vi "esdaq_demo.vi"() -> ()   [LabVIEW 2019]
panel:
  out "esdaqErrorOut":errorcluster
  out "DO_Array":bool[](array[boolean])
  in  "COM Status":bool
  in  "COM Port":refnum<visa-resource-name>
  in  "DIO_Array":T1(array[cluster])
  in  "AO_Array":T2(array[cluster])
  out "AI_Array":T3(array[cluster])
  # "ESDAQ-Data Acquisition System-13 DIO, 8 AI, 2 AO"
  # "Interactive Control Panel"
  # "https://github.com/enginsubasi/esdaqsys"
  # "https://github.com/enginsubasi/esdaqsys/wiki"
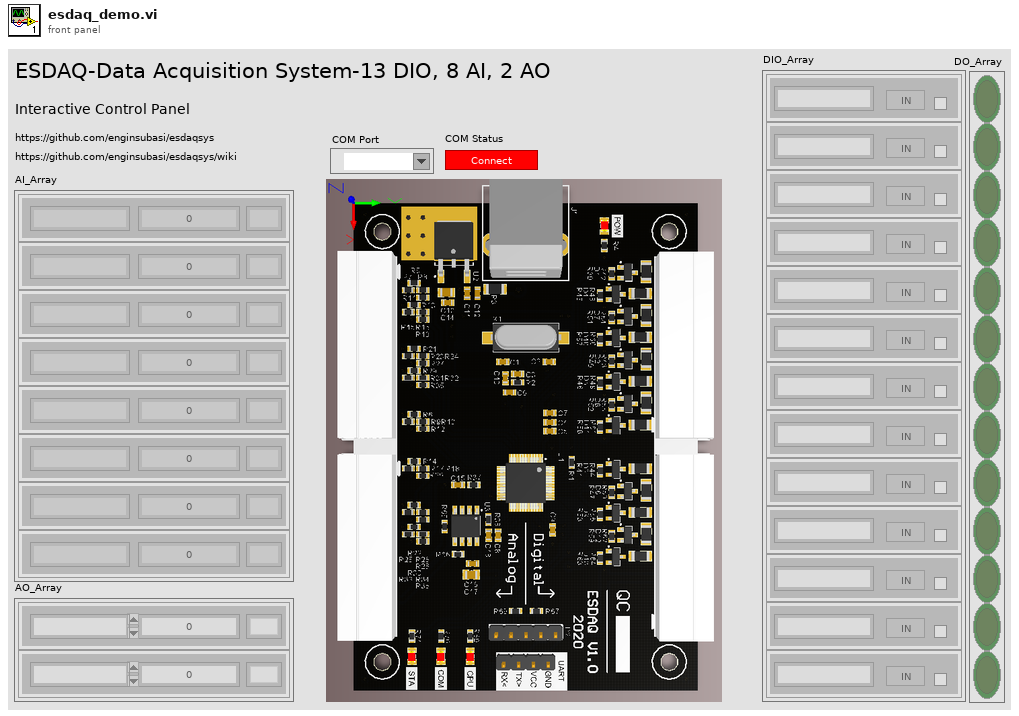
[diagram p1: front panel]
types:
  T1 = cluster{"Channel":string, "Direction":bool, "Drive":bool}[]
  T2 = cluster{"Value":u32, "Channel":string, "Unit":string}[]
  T3 = cluster{"Value":i32, "Channel":string, "Unit":string}[]
  T4 = cluster{"Value":i32, "Channel":string, "Unit":string}
  T5 = cluster{"Channel":bool, "Direction":bool, "Drive":bool}[]
  T6 = cluster{"Channel":string, "Direction":bool, "Drive":bool}
  T7 = cluster{"Value":bool, "Channel":bool, "Unit":bool}[]
  T8 = cluster{"Value":u32, "Channel":string, "Unit":string}
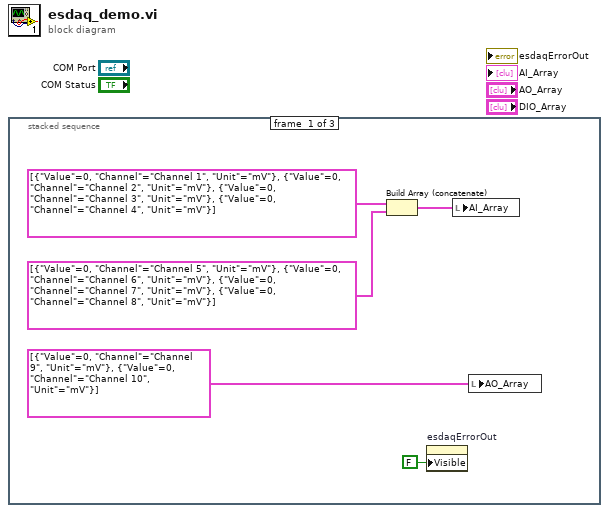
[diagram p0: block diagram]
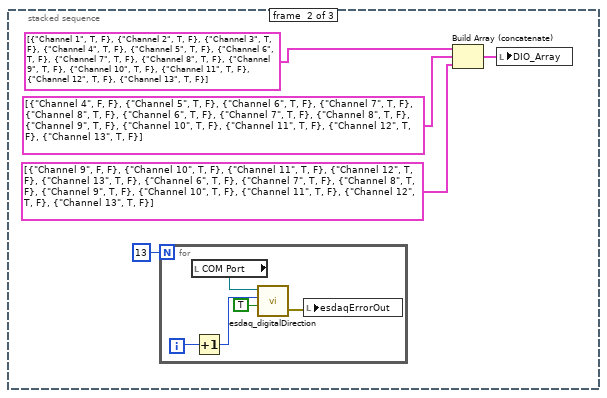
[diagram p2: hidden frame]
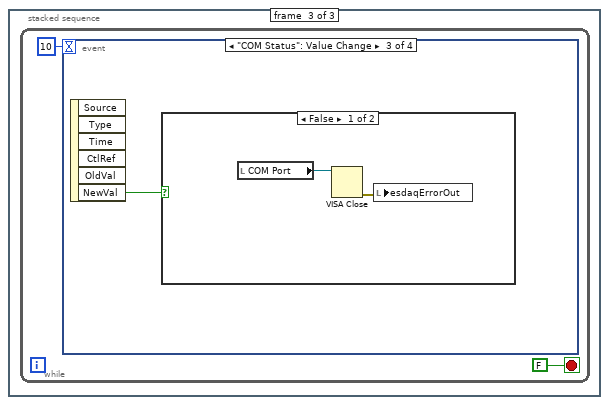
[diagram p3: hidden frame]
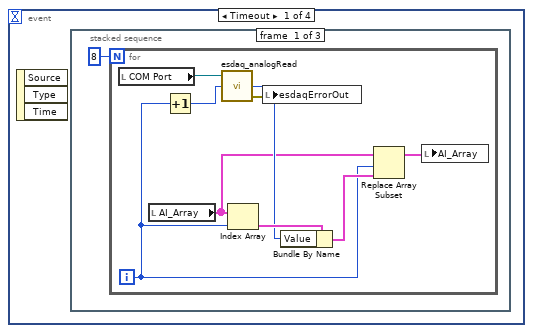
[diagram p4: hidden frame]
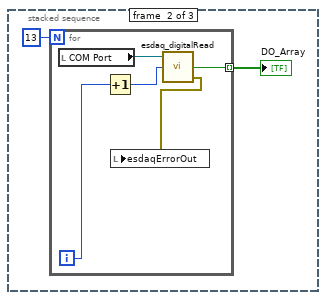
[diagram p5: hidden frame]
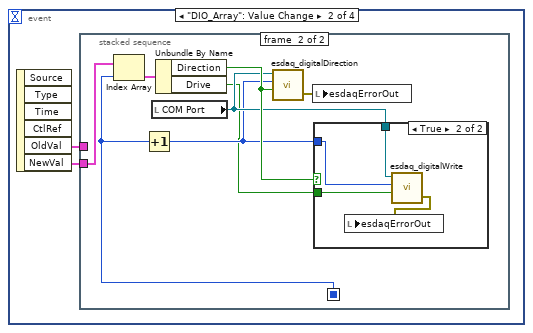
[diagram p7: hidden frame]
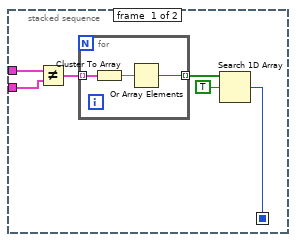
[diagram p8: hidden frame]
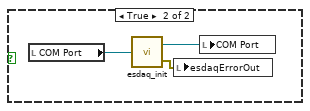
[diagram p10: hidden frame]
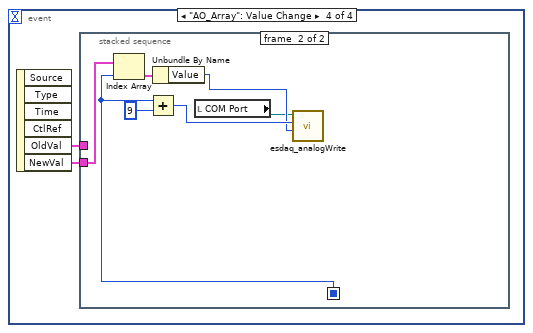
[diagram p11: hidden frame]
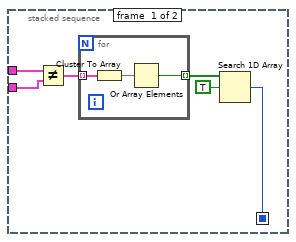
[diagram p12: hidden frame]
diagram:
  n1 = stacked-sequence {
    frame #0 {
      n2 = Build Array (concatenate)(T3 [{"Value"=0, "Channel"="Channel 1", "Unit"="mV"}, {"Value"=0, "Channel"="Channel 2", "Unit"="mV"}, {"Value"=0, "Channel"="Channel 3", "Unit"="mV"}, {"Value"=0, "Channel"="Channel 4", "Unit"="mV"}] ("AI_Array"), T3 [{"Value"=0, "Channel"="Channel 5", "Unit"="mV"}, {"Value"=0, "Channel"="Channel 6", "Unit"="mV"}, {"Value"=0, "Channel"="Channel 7", "Unit"="mV"}, {"Value"=0, "Channel"="Channel 8", "Unit"="mV"}] ("AI_Array")) -> (w3:T3)
      n3 = property on="esdaqErrorOut" class="Clust (strict)"("Visible"=FALSE) -> ()  [unwired: 2 in, 2 out]
      n4 = local write "AI_Array"(w3) -> ()
      n5 = local write "AO_Array"(T2 [{"Value"=0, "Channel"="Channel 9", "Unit"="mV"}, {"Value"=0, "Channel"="Channel 10", "Unit"="mV"}] ("AO_Array")) -> ()
    }
    frame #1 {
      n6 = for {
        N: 13 -> [_]
        i -> [w15]
        n7 = local read "COM Port"() -> (w12:refnum<visa-resource-name>)
        n8 = Increment(x=w15) -> (x+1=w14:i32)
        n9 = call "esdaq_digitalDirection.vi"("Value"=TRUE, "Channel"=w14, "esdaqPortInp"=w12) -> ("esdaqErrorOut"=w11:errorcluster)  [unwired: 1 in, 1 out]
        n10 = local write "esdaqErrorOut"(w11) -> ()
      }
      n11 = Build Array (concatenate)(T1 [{"Channel"="Channel 1", "Direction"=TRUE, "Drive"=FALSE}, {"Channel"="Channel 2", "Direction"=TRUE, "Drive"=FALSE}, {"Channel"="Channel 3", "Direction"=TRUE, "Drive"=FALSE}, {"Channel"="Channel 4", "Direction"=TRUE, "Drive"=FALSE}, {"Channel"="Channel 5", "Direction"=TRUE, "Drive"=FALSE}, {"Channel"="Channel 6", "Direction"=TRUE, "Drive"=FALSE}, {"Channel"="Channel 7", "Direction"=TRUE, "Drive"=FALSE}, {"Channel"="Channel 8", "Direction"=TRUE, "Drive"=FALSE}, {"Channel"="Channel 9", "Direction"=TRUE, "Drive"=FALSE}, {"Channel"="Channel 10", "Direction"=TRUE, "Drive"=FALSE}, {"Channel"="Channel 11", "Direction"=TRUE, "Drive"=FALSE}, {"Channel"="Channel 12", "Direction"=TRUE, "Drive"=FALSE}, {"Channel"="Channel 13", "Direction"=TRUE, "Drive"=FALSE}] ("DIO_Array"), T1 [{"Channel"="Channel 4", "Direction"=FALSE, "Drive"=FALSE}, {"Channel"="Channel 5", "Direction"=TRUE, "Drive"=FALSE}, {"Channel"="Channel 6", "Direction"=TRUE, "Drive"=FALSE}, {"Channel"="Channel 7", "Direction"=TRUE, "Drive"=FALSE}, {"Channel"="Channel 8", "Direction"=TRUE, "Drive"=FALSE}, {"Channel"="Channel 6", "Direction"=TRUE, "Drive"=FALSE}, {"Channel"="Channel 7", "Direction"=TRUE, "Drive"=FALSE}, {"Channel"="Channel 8", "Direction"=TRUE, "Drive"=FALSE}, {"Channel"="Channel 9", "Direction"=TRUE, "Drive"=FALSE}, {"Channel"="Channel 10", "Direction"=TRUE, "Drive"=FALSE}, {"Channel"="Channel 11", "Direction"=TRUE, "Drive"=FALSE}, {"Channel"="Channel 12", "Direction"=TRUE, "Drive"=FALSE}, {"Channel"="Channel 13", "Direction"=TRUE, "Drive"=FALSE}] ("DIO_Array"), T1 [{"Channel"="Channel 9", "Direction"=FALSE, "Drive"=FALSE}, {"Channel"="Channel 10", "Direction"=TRUE, "Drive"=FALSE}, {"Channel"="Channel 11", "Direction"=TRUE, "Drive"=FALSE}, {"Channel"="Channel 12", "Direction"=TRUE, "Drive"=FALSE}, {"Channel"="Channel 13", "Direction"=TRUE, "Drive"=FALSE}, {"Channel"="Channel 6", "Direction"=TRUE, "Drive"=FALSE}, {"Channel"="Channel 7", "Direction"=TRUE, "Drive"=FALSE}, {"Channel"="Channel 8", "Direction"=TRUE, "Drive"=FALSE}, {"Channel"="Channel 9", "Direction"=TRUE, "Drive"=FALSE}, {"Channel"="Channel 10", "Direction"=TRUE, "Drive"=FALSE}, {"Channel"="Channel 11", "Direction"=TRUE, "Drive"=FALSE}, {"Channel"="Channel 12", "Direction"=TRUE, "Drive"=FALSE}, {"Channel"="Channel 13", "Direction"=TRUE, "Drive"=FALSE}] ("DIO_Array")) -> (w7:T1)
      n12 = local write "DIO_Array"(w7) -> ()
    }
    frame #2 {
      n13 = while {
        stop <- FALSE stop-if-true
        n14 = event shown="[2] \"COM Status\": Value Change" {
          selector: _ -> [_ _ _ _]
          dyn-events: _ -> [_ _ _ _]
          timeout: 10 -> [_ _ _ _]
          event Timeout {
            n15 = event-data() -> ()  [unwired: 1 in, 3 out]
            n16 = stacked-sequence {
              frame #0 {
                n17 = for {
                  N: 8 -> [_]
                  i -> [w20]
                  n18 = local read "COM Port"() -> (w27:refnum<visa-resource-name>)
                  n19 = local read "AI_Array"() -> (w23:T3)
                  n20 = Increment(x=w20) -> (x+1=w26:i32)
                  n21 = call "esdaq_analogRead.vi"("Channel"=w26, "esdaqPortInp"=w27) -> ("esdaqErrorOut"=w19:errorcluster, "value"=w24:i32)  [unwired: 1 in, 1 out]
                  n22 = Index Array(array=w23, index=w20) -> (element=w25:T4)
                  n23 = local write "esdaqErrorOut"(w19) -> ()
                  n24 = Bundle By Name(cluster=w25, "Value"=w24) -> (w22:T4)
                  n25 = Replace Array Subset(array=w23, new element=w22, index=w20) -> (w21:T3)
                  n26 = local write "AI_Array"(w21) -> ()
                }
              }
              frame #1 {
                n27 = for {
                  N: 13 -> [_]
                  tunnel: [w31] -> w28 mode=indexing
                  i -> [w34]
                  n28 = local read "COM Port"() -> (w33:refnum<visa-resource-name>)
                  n29 = Increment(x=w34) -> (x+1=w32:i32)
                  n30 = call "esdaq_digitalRead.vi"("Channel"=w32, "esdaqPortInp"=w33) -> ("esdaqErrorOut"=w30:errorcluster, "Value"=w31:bool)  [unwired: 1 in, 1 out]
                  n31 = local write "esdaqErrorOut"(w30) -> ()
                }
                "DO_Array" <- w28
              }
              frame #2 {
              }
            }
          }
          event "DIO_Array": Value Change {
            n32 = event-data() -> ("OldVal"=w36:T1, "NewVal"=w35:T1)  [unwired: 1 in, 4 out]
            n33 = stacked-sequence {
              seq-local: [w37 _] -> [_ w51]
              tunnel: w36 -> [w42 _]
              tunnel: w35 -> [w41 w53]
              frame #0 {
                n34 = Not Equal?(x=w42, y=w41) -> (x != y?=w40:T5)
                n35 = for {
                  tunnel: w40 -> [w45] mode=indexing
                  tunnel: [w43] -> w39 mode=indexing
                  n36 = Cluster To Array(cluster=w45) -> (array=w44:bool[])
                  n37 = Or Array Elements(Boolean array=w44) -> (logical OR=w43:bool)
                }
                n38 = Search 1D Array(1D array=w39, element=TRUE) -> (index of element=w37:i32)  [unwired: 1 in]
              }
              frame #1 {
                n39 = Index Array(array=w53, index=w51) -> (element=w52:T6)
                n40 = Increment(x=w51) -> (x+1=w48:i32)
                n41 = local read "COM Port"() -> (w49:refnum<visa-resource-name>)
                n42 = Unbundle By Name(w52) -> ("Direction"=w50:bool, "Drive"=w47:bool)
                n43 = call "esdaq_digitalDirection.vi"("Value"=w50, "Channel"=w48, "esdaqPortInp"=w49) -> ("esdaqErrorOut"=w46:errorcluster)  [unwired: 1 in, 1 out]
                n44 = local write "esdaqErrorOut"(w46) -> ()
                n45 = case shown="True" w50 {
                  tunnel: w49 -> [_ w57]
                  tunnel: w48 -> [_ w56]
                  tunnel: w47 -> [_ w55]
                  frame False {
                  }
                  frame True {
                    n46 = call "esdaq_digitalWrite.vi"("Value"=w55, "Channel"=w56, "esdaqPortInp"=w57) -> ("esdaqErrorOut"=w54:errorcluster)  [unwired: 1 in, 1 out]
                    n47 = local write "esdaqErrorOut"(w54) -> ()
                  }
                }
              }
            }
          }
          event "COM Status": Value Change {
            n48 = event-data() -> ("NewVal"=w58:bool)  [unwired: 1 in, 5 out]
            n49 = case shown="False" w58 {
              frame False {
                n50 = local read "COM Port"() -> (w60:refnum<visa-resource-name>)
                n51 = VISA Close(VISA resource name=w60) -> (error out=w59:errorcluster)  [unwired: 1 in]
                n52 = local write "esdaqErrorOut"(w59) -> ()
              }
              frame True {
                n53 = local read "COM Port"() -> (w62:refnum<visa-resource-name>)
                n54 = call "esdaq_init.vi"("esdaqPortInp"=w62) -> ("esdaqPortOut"=w63:refnum<visa-resource-name>, "esdaqErrorOut"=w61:errorcluster)
                n55 = local write "esdaqErrorOut"(w61) -> ()
                n56 = local write "COM Port"(w63) -> ()
              }
            }
          }
          event "AO_Array": Value Change {
            n57 = event-data() -> ("OldVal"=w65:T2, "NewVal"=w64:T2)  [unwired: 1 in, 4 out]
            n58 = stacked-sequence {
              seq-local: [w66 _] -> [_ w79]
              tunnel: w65 -> [w71 _]
              tunnel: w64 -> [w70 w81]
              frame #0 {
                n59 = Not Equal?(x=w71, y=w70) -> (x != y?=w69:T7)
                n60 = for {
                  tunnel: w69 -> [w74] mode=indexing
                  tunnel: [w72] -> w68 mode=indexing
                  n61 = Cluster To Array(cluster=w74) -> (array=w73:bool[])
                  n62 = Or Array Elements(Boolean array=w73) -> (logical OR=w72:bool)
                }
                n63 = Search 1D Array(1D array=w68, element=TRUE) -> (index of element=w66:i32)  [unwired: 1 in]
              }
              frame #1 {
                n64 = Index Array(array=w81, index=w79) -> (element=w80:T8)
                n65 = Add(x=w79, y=9) -> (x+y=w77:i32)
                n66 = Unbundle By Name(w80) -> ("Value"=w76:u32)
                n67 = local read "COM Port"() -> (w75:refnum<visa-resource-name>)
                n68 = call "esdaq_analogWrite.vi"("Value"=w76, "Channel"=w77, "esdaqPortInp"=w75) -> ()  [unwired: 1 in, 2 out]
              }
            }
          }
        }
      }
    }
  }
